vi "Valve Conversion (SubVI).vi"(2 "Valve Array In":dbl[](array[numeric]), 4 "Button Array":dbl[](array[numeric])) -> (0 "LED Array":bool[](array[boolean]), 1 "Comparison Out":bool[](array[boolean]), 3 "Ignitor State":dbl)   [LabVIEW 2020]
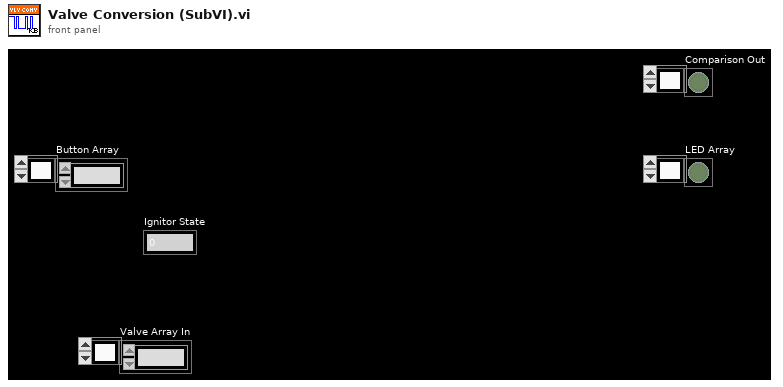
[diagram p1: front panel]
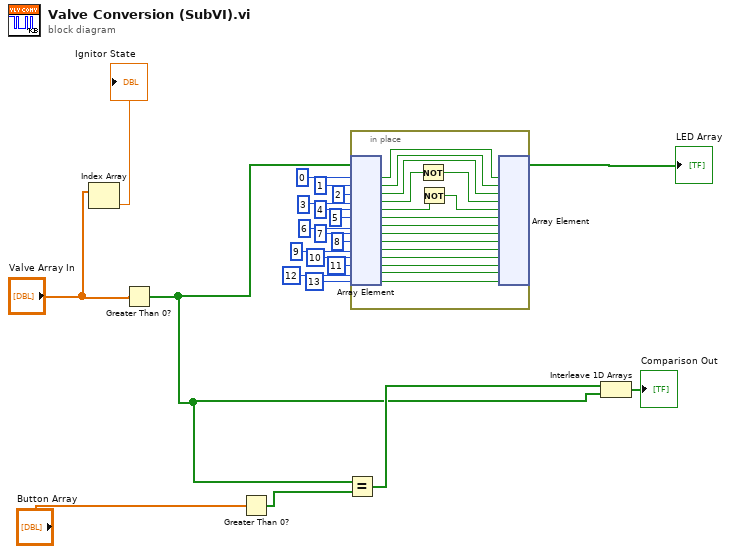
[diagram p0: block diagram]
diagram:
  n1 = Index Array(array="Valve Array In") -> (element=→"Ignitor State":dbl)  [unwired: 1 in]
  n2 = Greater Than 0?(x="Valve Array In") -> (x > 0?=w1:bool[])
  n3 = Greater Than 0?(x="Button Array") -> (x > 0?=w4:bool[])
  n4 = Equal?(x=w1, y=w4) -> (x = y?=w2:bool[])
  n5 = in-place {
    n6 = in-place-array #1(w1, 0, 1, 2, 3, 4, 5, 6, 7, 8, 9, 10, 11, 12, 13) -> (w38:bool, w37:bool, w36:bool, w35:bool, w33:bool, w31:bool, w30:bool, w29:bool, w28:bool, w27:bool, w26:bool, w25:bool, w24:bool, w23:bool)
    n7 = Not(x=w35) -> (.not. x?=w34:bool)
    n8 = Not(x=w33) -> (.not. x?=w32:bool)
    n9 = in-place-array #1(w38, w37, w36, w34, w32, w31, w30, w29, w28, w27, w26, w25, w24, w23) -> (→"LED Array":bool[])  [unwired: 14 out]
  }
  n10 = Interleave 1D Arrays(w2, w1) -> (→"Comparison Out":bool[])
